vi "Create Wrapper for Code Module - Multiple Convertervi.vi"(11 "error in":errorcluster) -> (15 "error out":errorcluster)   [LabVIEW 2021, in "Converter.lvlib"]
uses:
  Converter.lvlib
  <vilib>/Utility/miscctls.llb/LVPointTypeDef.ctl
  <vilib>/Utility/traverseref.llb/TRef TravTarget.ctl
  <vilib>/Utility/traverseref.llb/VI Scripting - Traverse.lvlib
  Converter Reusables/Converter Reusables.lvlib
  Path Functions/Path Functions.lvlib
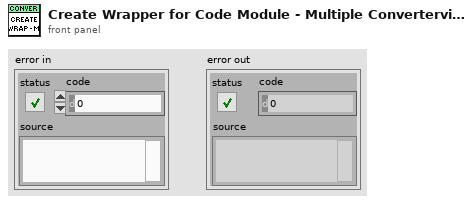
[diagram p1: front panel]
types:
  T1 = typedef "TRef TravTarget.ctl" = enum16{"FP", "BD", "Other"}
  T2 = typedef "LVPointTypeDef.ctl" = cluster{"Horizontal":i16, "Vertical":i16}
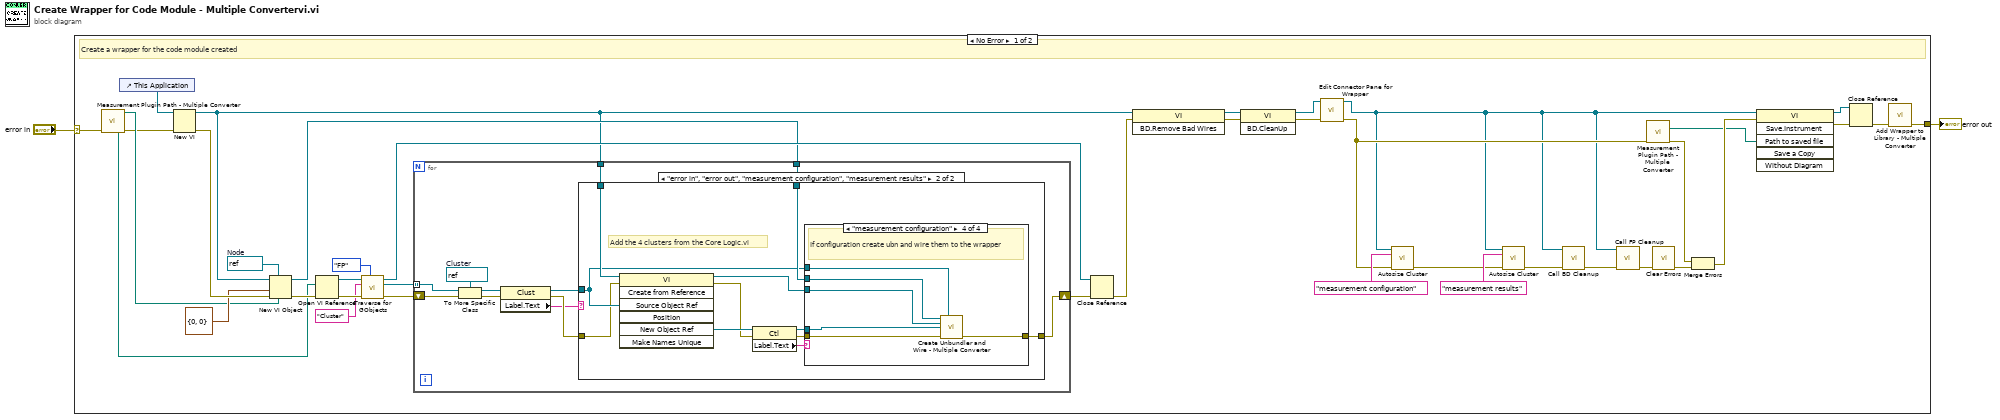
[diagram p0: block diagram]
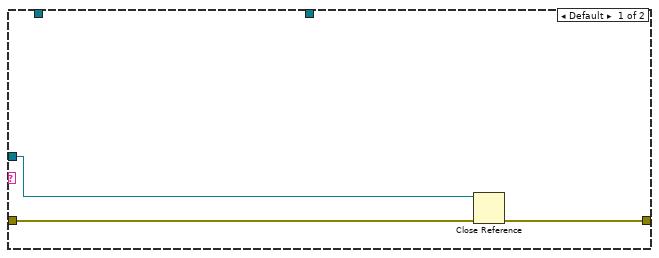
[diagram p2: hidden frame]
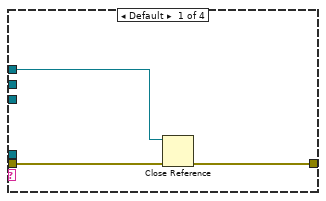
[diagram p3: hidden frame]
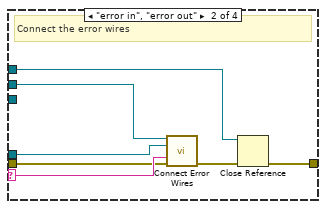
[diagram p4: hidden frame]
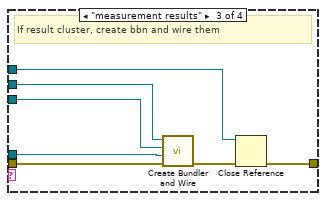
[diagram p5: hidden frame]
diagram:
  n1 = case shown="No Error" "error in" {
    selector: "error in" -> [w14 w91]
    tunnel: [w9 w91] -> w2
    frame No Error {
      w42 = refnum<vi> refnum  # Node
      # "Create a wrapper for the code module created"
      n2 = call "Measurement Plugin Path - Multiple Converter.vi"("error in"=w14) -> ("new code module"=w16:path, "logic vi path"=w15:path, "error out"=w13:errorcluster)  [unwired: 2 in, 10 out]
      n3 = control-ref of="This Application"() -> (w27:refnum<vi>)
      n4 = New VI(8:w13, 11:w27) -> (0:w41:errorcluster, 3:w26:refnum<vi>)  [unwired: 5 in]
      n5 = New VI Object(vi object class=w42, owner refnum=w26, position/next to=T2 {"Horizontal"=0, "Vertical"=0} ("location"), 6:w16, 8:w41) -> (object refnum=w28:refnum<vi>, 0:w37:errorcluster)  [unwired: 3 in]
      n6 = Open VI Reference(vi path=w15, error in (no error)=w37) -> (vi reference=w33:refnum<vi>, error out=w36:errorcluster)  [unwired: 4 in]
      n7 = call <vilib>:"Traverse for GObjects.vi"("Traverse Target"=TRef_TravTarget."FP", "error in (no error)"=w36, "Class Name"="Cluster", "VI Refnum"=w33) -> ("error out"=w34:errorcluster, "References"=w31:refnum<vi>[], "dup VI Refnum"=w30:refnum<vi>)  [unwired: 4 in, 1 out]
      n8 = for {
        shift-right: [w49] -> w32
        shift-left: w34 -> [w52]
        tunnel: w31 -> [w48] mode=indexing
        tunnel: w26 -> [w51]
        tunnel: w28 -> [w50]
        w53 = refnum<vi> refnum  # Cluster
        n9 = To More Specific Class(target class=w53, reference=w48, error in=w52) -> (specific class reference=w45:refnum<vi>, error out=w47:errorcluster)
        n10 = property class="Clust"(reference=w45, error in=w47) -> (reference out=w44:refnum<vi>, error out=w46:errorcluster, "Label.Text"=w43:string)
        n11 = case shown="\"error in\", \"error out\", \"measurement configuration\", \"measurement results\"" w43 {
          tunnel: w51 -> [_ w67]
          tunnel: w50 -> [_ w61]
          tunnel: [w55 w60] -> w49
          tunnel: w44 -> [w54 w58]
          tunnel: w46 -> [w56 w57]
          frame Default {
            n12 = Close Reference(reference=w54, error in (no error)=w56) -> (error out=w55:errorcluster)
          }
          frame "error in", "error out", "measurement configuration", "measurement results" {
            # "Add the 4 clusters from the Core Logic.vi"
            n13 = invoke class="VI" method="Create from Reference"(reference=w67, error in=w57, "Source Object Ref"=w58) -> (reference out=w62:refnum<vi>, error out=w65:errorcluster, "New Object Ref"=w66:refnum<vi>)  [unwired: 4 in, 4 out]
            n14 = property class="Ctl"(reference=w66, error in=w65) -> (reference out=w59:refnum<vi>, error out=w64:errorcluster, "Label.Text"=w63:string)
            n15 = case shown="\"measurement configuration\"" w63 {
              selector: w63 -> [_ w76 _ _]
              tunnel: w64 -> [w70 w73 w84 w86]
              tunnel: w62 -> [_ _ w83 w87]
              tunnel: w61 -> [_ w77 w82 w88]
              tunnel: [w68 w72 w80 w90] -> w60
              tunnel: w58 -> [w69 w71 w79 w89]
              tunnel: w59 -> [_ w74 w78 w85]
              frame Default {
                n16 = Close Reference(reference=w69, error in (no error)=w70) -> (error out=w68:errorcluster)
              }
              frame "error in", "error out" {
                # "Connect the error wires"
                n17 = call "Connect Error Wires.vi"("node in"=w77, "new object ref"=w74, "string"=w76, "error in"=w73) -> ("error out"=w75:errorcluster)  [unwired: 11 in]
                n18 = Close Reference(reference=w71, error in (no error)=w75) -> (error out=w72:errorcluster)
              }
              frame "measurement results" {
                # "If result cluster, create bbn and wire them"
                n19 = call "Create Bundler and Wire.vi"("error in"=w84, "new object ref"=w78, "vi refnum"=w83, "node ref"=w82) -> ("error out"=w81:errorcluster)  [unwired: 7 in]
                n20 = Close Reference(reference=w79, error in (no error)=w81) -> (error out=w80:errorcluster)
              }
              frame "measurement configuration" {
                # "If configuration create ubn and wire them to the wrapper"
                n21 = call "Create Unbundler and Wire - Multiple Converter.vi"("node in"=w88, "clust refnum"=w89, "vi refnum"=w87, "new object ref"=w85, "error in"=w86) -> ("error out"=w90:errorcluster)  [unwired: 10 in]
              }
            }
          }
        }
      }
      n22 = Close Reference(reference=w30, error in (no error)=w32) -> (error out=w23:errorcluster)
      n23 = invoke class="VI" method="BD.Remove Bad Wires"(reference=w26, error in=w23) -> (reference out=w25:refnum<vi>, error out=w24:errorcluster)  [unwired: 1 in, 1 out]
      n24 = invoke class="VI" method="BD.CleanUp"(reference=w25, error in=w24) -> (reference out=w18:refnum<vi>, error out=w17:errorcluster)  [unwired: 1 in, 1 out]
      n25 = call "Edit Connector Pane for Wrapper.vi"("vi reference in"=w18, "error in"=w17) -> ("vi reference out"=w3:refnum<vi>, "error out"=w6:errorcluster)  [unwired: 12 in]
      n26 = call "Autosize Cluster.vi"("vi refnum"=w3, "name"="measurement configuration" ("name/order"), "error in"=w6) -> ("error out"=w5:errorcluster)  [unwired: 12 in]
      n27 = call "Autosize Cluster.vi"("vi refnum"=w3, "name"="measurement results" ("name/order"), "error in"=w5) -> ("error out"=w4:errorcluster)  [unwired: 12 in]
      n28 = call "Call BD Cleanup.vi"("vi"=w3, "error in"=w4) -> ("error out"=w22:errorcluster)  [unwired: 13 in]
      n29 = call "Call FP Cleanup.vi"("vi"=w3, "error in"=w22) -> ("error out"=w21:errorcluster)  [unwired: 13 in]
      n30 = call "Measurement Plugin Path - Multiple Converter.vi"("error in"=w6) -> ("wrapper path"=w12:path, "error out"=w11:errorcluster)  [unwired: 2 in, 11 out]
      n31 = call <vilib>:"Clear Errors.vi"("error in (no error)"=w21) -> ("error out"=w20:errorcluster)  [unwired: 5 in, 1 out]
      n32 = Merge Errors(w11, w20) -> (w19:errorcluster)
      n33 = invoke class="VI" method="Save.Instrument"(reference=w3, error in=w19, "Path to saved file"=w12) -> (reference out=w38:refnum<vi>, error out=w39:errorcluster)  [unwired: 3 in, 4 out]
      n34 = Close Reference(reference=w38, error in (no error)=w39) -> (error out=w10:errorcluster)
      n35 = call "Add Wrapper to Library - Multiple Converter.vi"("error in"=w10) -> ("error out"=w9:errorcluster)  [unwired: 14 in]
    }
    frame Error {
    }
  }
  "error out" <- w2
